vi "Czy nowa wartość współrzędnych.vi"(8 "b":dbl, 9 "a":dbl, 10 "szerokość geograficzna":dbl, 11 "Długość geograficzna":dbl) -> (0 "Czy nowa wartość":bool, 2 "Położenie":cluster{"X/E [m]":dbl, "Y/N [m]":dbl}, 3 "Położenie \nrobota  UTM":T1)   [LabVIEW 2012, in "Biblioteka moduł map v3.lvlib" / "Konwersja wsp.lvlib" / "UTM.lvlib"]
uses:
  UTM.lvlib
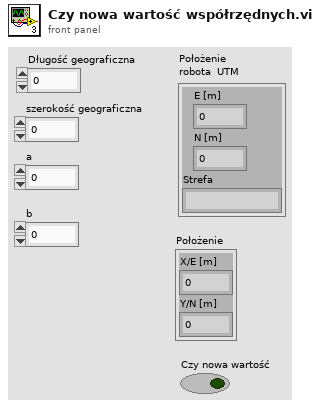
[diagram p1: front panel]
types:
  T1 = cluster{"E [m]":ext, "N [m]":ext, "Strefa":string}
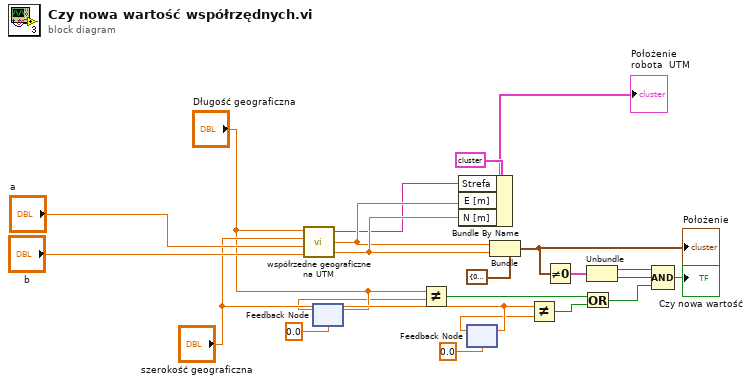
[diagram p0: block diagram]
diagram:
  n1 = call "współrzedne geograficzne na UTM.vi"("Położenie robota - długość geograficzna"="Długość geograficzna", "Położenie robota - szerokość geograficzna"="szerokość geograficzna", "a"="a", "b"="b") -> ("Strefa"=w20:string, "E"=w21:ext, "N"=w22:ext)  [unwired: 2 in]
  n2 = feedback #1(0.0 ("X")) -> (w13:dbl)
  n3 = feedback-in #1("Długość geograficzna") -> ()
  n4 = Not Equal?(x="Długość geograficzna", y=w13) -> (x != y?=w7:bool)
  n5 = Bundle By Name(cluster=T1 {"E [m]"=0.0, "N [m]"=0.0, "Strefa"=""} ("Położenie \nrobota  UTM"), "Strefa"=w20, "E [m]"=w21, "N [m]"=w22) -> (→"Położenie \nrobota  UTM":T1)
  n6 = feedback #2(0.0 ("X")) -> (w11:dbl)
  n7 = feedback-in #2("szerokość geograficzna") -> ()
  n8 = Bundle(cluster=cluster{"X [m]":dbl, "Y [m]":dbl} {"X [m]"=0.0, "Y [m]"=0.0}, "X [m]"=w21, "Y [m]"=w22) -> (w2:cluster{"X [m]":dbl, "Y [m]":dbl})
  "Położenie" <- w2
  n9 = Not Equal?(x="szerokość geograficzna", y=w11) -> (x != y?=w8:bool)
  n10 = Not Equal To 0?(x=w2) -> (x != 0?=w3:cluster{"X [m]":bool, "Y [m]":bool})
  n11 = Or(x=w7, y=w8) -> (x .or. y?=w9:bool)
  n12 = Unbundle(w3) -> ("X [m]"=w4:bool, "Y [m]"=w5:bool)
  n13 = Compound Arithmetic op=AND(w4, w5, w9) -> (→"Czy nowa wartość":bool)
